vi "Test.vi"() -> ()   [LabVIEW 2020]
uses:
  Support/Controls/Cmd_Mouse Popup.ctl
  <vilib>/Utility/NIReport.llb/Report Type.ctl
  <vilib>/Utility/NIReport.llb/NI_report.lvclass
  <vilib>/Utility/NIReport.llb/Excel/NI_Excel.lvclass
  <vilib>/Utility/NIReport.llb/NI_ReportGenerationCore.lvlib
panel:
  in  "확인 버튼":bool
  in  "정지":bool
  in  "테이블 컨트롤":string[][](table)
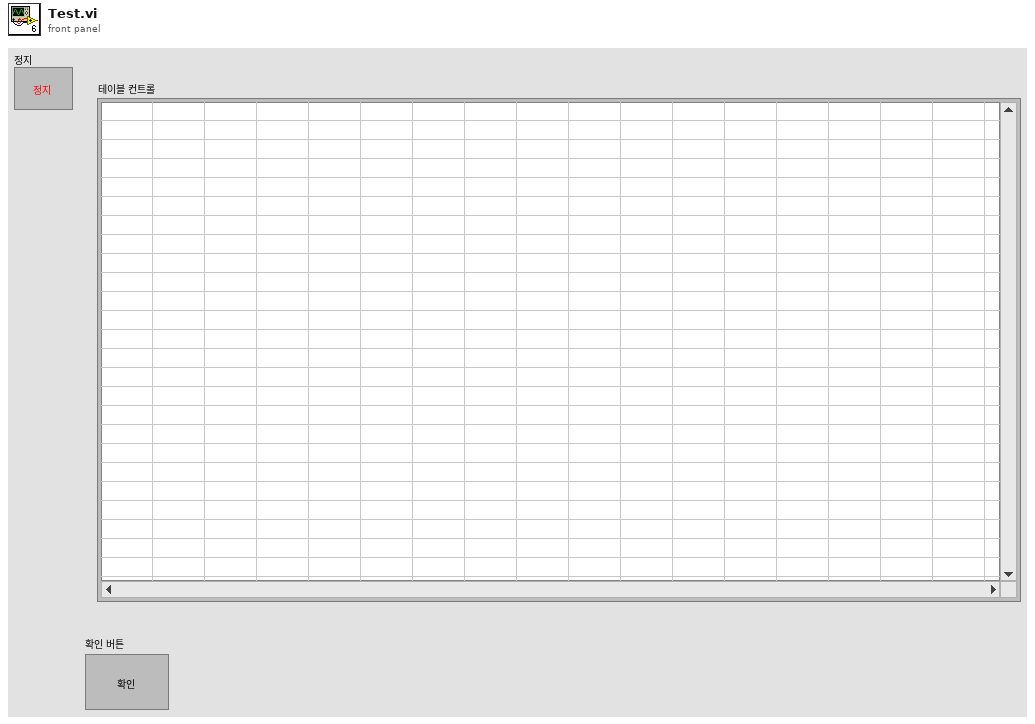
[diagram p1: front panel]
types:
  T1 = typedef "Cmd_Mouse Popup.ctl" = enum16{"활성화", "메뉴선택"}
  T2 = typedef "NI_ReportGenerationCore.lvlib/Report Type.ctl" = enum16{"HTML", "Word", "Excel"}
  T3 = enum16{"maximized", "minimized", "normal", "no change"}
  T4 = cluster{"Shift":bool, "Ctrl":bool, "Alt":bool, "Cmd":bool, "Opt":bool}
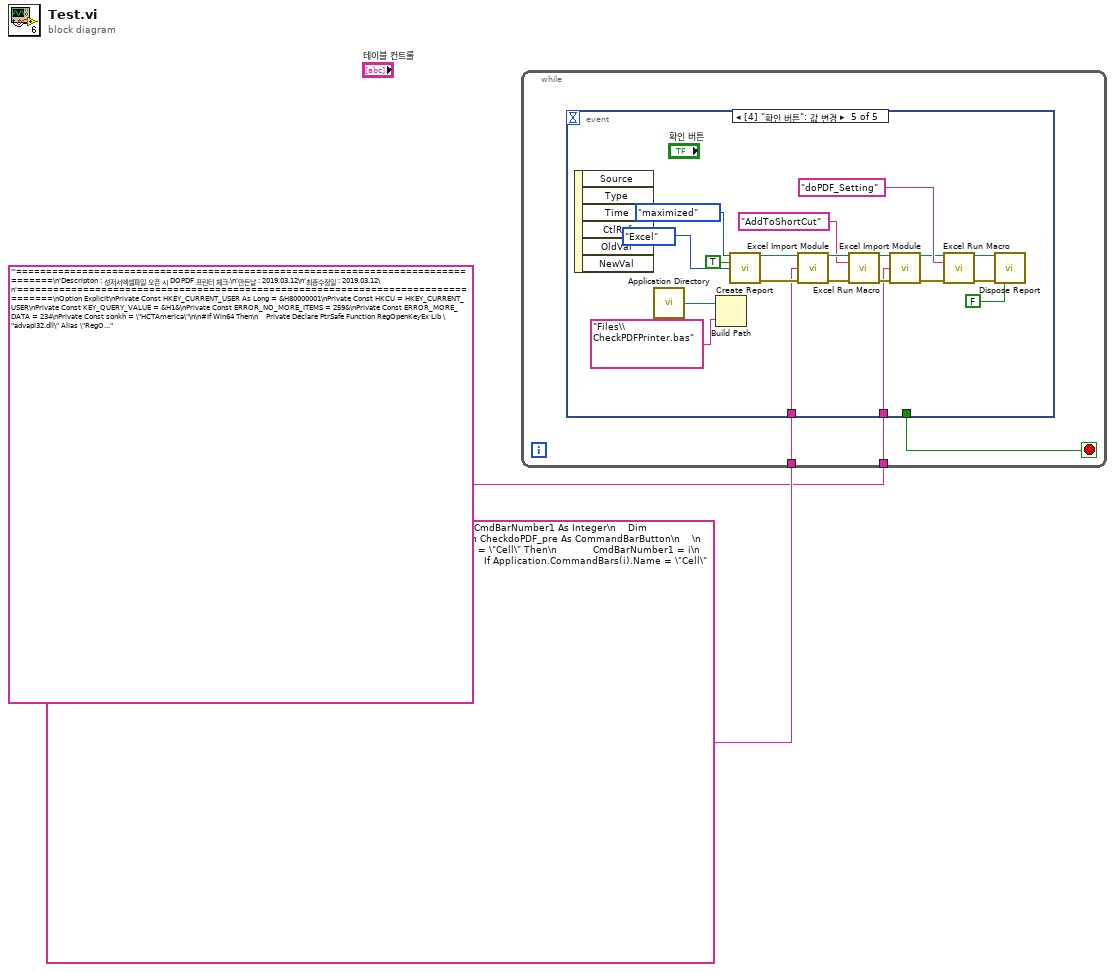
[diagram p0: block diagram]
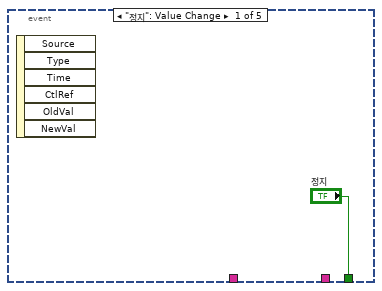
[diagram p2: hidden frame]
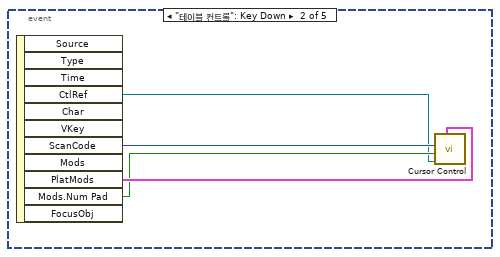
[diagram p3: hidden frame]
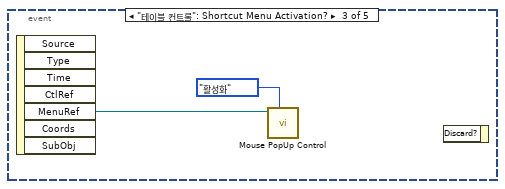
[diagram p4: hidden frame]
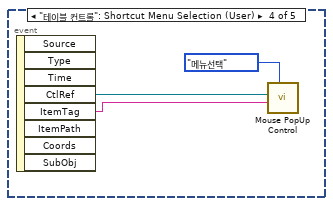
[diagram p5: hidden frame]
diagram:
  n1 = while {
    tunnel: "Sub AddToShortCut()\n\n    Dim i As Integer\n    Dim CmdBarNumber As Integer\n    Dim CmdBarNumber1 As Integer\n    Dim CmdBarNumber2 As Integer\n    Dim CheckdoPDF_preview As CommandBarButton\n    Dim CheckdoPDF_pre As CommandBarButton\n    \n    For i = 1 To Application.CommandBars.Count\n        If Application.CommandBars(i).Name = \"Cell\" Then\n            CmdBarNumber1 = i\n            Exit For\n        End If\n    Next\n\n    For i = 1 + i To Application.CommandBars.Count\n        If Application.CommandBars(i).Name = \"Cell\" Then\n            CmdBarNumber2 = i\n            Exit For\n        End If\n    Next\n\n    For i = 0 To 1\n\n        If i = 0 Then\n            CmdBarNumber = CmdBarNumber1\n        Else\n            CmdBarNumber = CmdBarNumber2\n        End If\n\n        With Application.CommandBars(CmdBarNumber)\n\n            .Reset\n            Set CheckdoPDF_preview = .Controls.Add(Type:=msoControlButton, Before:=8, Temporary:=True)\n            Set CheckdoPDF_pre = .Controls.Add(Type:=msoControlButton, Before:=9, Temporary:=True)\n            .Controls(10).BeginGroup = True\n\n        End With\n\n      \n        With CheckdoPDF_preview\n            .Caption = \"성적서출력확인(Preview)\"\n            .OnAction = \"xlPageBreakPreview_on\"\n            .FaceId = 487\n        End With\n        \n        With CheckdoPDF_pre\n            .Caption = \"성적서출력확인완료(업로드가능)\"\n            .OnAction = \"UpdatePreviewcheck\"\n            .FaceId = 487\n        End With\n        \n    Next\nEnd Sub\n" -> [w4]
    tunnel: "'==================================================================================\n'Descripton : 성저서엑셀파일 오픈 시 DOPDF 프린터 체크.\n'만든날 : 2019.03.12\n'최종수정일 : 2019.03.12\n'==================================================================================\nOption Explicit\nPrivate Const HKEY_CURRENT_USER As Long = &H80000001\nPrivate Const HKCU = HKEY_CURRENT_USER\nPrivate Const KEY_QUERY_VALUE = &H1&\nPrivate Const ERROR_NO_MORE_ITEMS = 259&\nPrivate Const ERROR_MORE_DATA = 234\nPrivate Const sonkh = \"HCTAmerica\"\n\n#If Win64 Then\n    Private Declare PtrSafe Function RegOpenKeyEx Lib \"advapi32.dll\" Alias \"RegOpenKeyExA\" ( _\n         ByVal hKey As LongPtr, _\n         ByVal lpSubKey As String, _\n         ByVal ulOptions As Long, _\n         ByVal samDesired As Long, _\n         phkResult As LongPtr) As Long\n  \n    Private Declare PtrSafe Function RegEnumValue Lib \"advapi32.dll\" Alias \"RegEnumValueA\" ( _\n          ByVal hKey As LongPtr, ByVal dwIndex As Long, ByVal lpValueName As String, _\n          lpcbValueName As Long, ByVal lpReserved As Long, lpType As Long, _\n          lpData As Byte, lpcbData As Long) As Long\n         \n    Private Declare PtrSafe Function RegCloseKey Lib \"advapi32.dll\" ( _\n         ByVal hKey As LongPtr) As Long\n     \n#Else\n    Private Declare Function RegOpenKeyEx Lib \"advapi32\" _\n        Alias \"RegOpenKeyExA\" ( _\n        ByVal hKey As Long, _\n        ByVal lpSubKey As String, _\n        ByVal ulOptions As Long, _\n        ByVal samDesired As Long, _\n        phkResult As Long) As Long\n    \n    Private Declare Function RegEnumValue Lib \"advapi32.dll\" _\n        Alias \"RegEnumValueA\" ( _\n        ByVal hKey As Long, _\n        ByVal dwIndex As Long, _\n        ByVal lpValueName As String, _\n        lpcbValueName As Long, _\n        ByVal lpReserved As Long, _\n        lpType As Long, _\n        lpData As Byte, _\n        lpcbData As Long) As Long\n    \n    Private Declare Function RegCloseKey Lib \"advapi32.dll\" ( _\n        ByVal hKey As Long) As Long\n    \n#End If\n    \nPrivate Function Crypt_EXcel(texti, salt) As String\n    Dim X1 As Long\n    Dim T, TT As Long\n    Dim G, sana As Long\n    Dim Crypted As String\n    \n  On Error Resume Next\n\n  For T = 1 To Len(salt)\n    sana = Asc(Mid(salt, T, 1))\n    X1 = X1 + sana\n  Next\n\n  X1 = Int((X1 * 0.1) / 6)\n  salt = X1\n  G = 0\n\n  For TT = 1 To Len(texti)\n    sana = Asc(Mid(texti, TT, 1))\n\n    G = G + 1\n\n    If G = 6 Then G = 0\n\n    X1 = 0\n\n    If G = 0 Then X1 = sana - (salt - 2)\n    If G = 1 Then X1 = sana + (salt - 5)\n    If G = 2 Then X1 = sana - (salt - 4)\n    If G = 3 Then X1 = sana + (salt - 2)\n    If G = 4 Then X1 = sana - (salt - 3)\n    If G = 5 Then X1 = sana + (salt - 5)\n\n    X1 = X1 + G\n\n    Crypted = Crypted & Chr(X1)\n\n  Next\n\n  Crypt_EXcel = Crypted\n\nEnd Function\nPrivate Function GetPrinterFullNames() As String()\nDim Printers() As String ' array of names to be returned\nDim PNdx As Long    ' index into Printers()\n'Dim hKey As Long    ' registry key handle\nDim Res As Long     ' result of API calls\nDim Ndx As Long     ' index for RegEnumValue\nDim ValueName As String ' name of each value in the printer key\nDim ValueNameLen As Long    ' length of ValueName\nDim DataType As Long        ' registry value data type\nDim ValueValue() As Byte    ' byte array of registry value value\nDim ValueValueS As String   ' ValueValue converted to String\nDim CommaPos As Long        ' position of comma character in ValueValue\nDim ColonPos As Long        ' position of colon character in ValueValue\nDim M As Long               ' string index\n\n#If Win64 Then\n    Dim L As LongPtr, hKey As LongPtr\n#Else\n    Dim L As Long, hKey As Long\n#End If\n\n' registry key in HCKU listing printers\nConst PRINTER_KEY = \"Software\\Microsoft\\Windows NT\\CurrentVersion\\Devices\"\n\nPNdx = 0\nNdx = 0\n' assume printer name is less than 256 characters\nValueName = String$(256, Chr(0))\nValueNameLen = 255\n' assume the port name is less than 1000 characters\nReDim ValueValue(0 To 999)\n' assume there are less than 1000 printers installed\nReDim Printers(1 To 1000)\n\n' open the key whose values enumerate installed printers\nRes = RegOpenKeyEx(HKCU, PRINTER_KEY, 0&, _\n    KEY_QUERY_VALUE, hKey)\n' start enumeration loop of printers\nRes = RegEnumValue(hKey, Ndx, ValueName, _\n    ValueNameLen, 0&, DataType, ValueValue(0), 1000)\n' loop until all values have been enumerated\nDo Until Res = ERROR_NO_MORE_ITEMS\n    M = InStr(1, ValueName, Chr(0))\n    If M > 1 Then\n        ' clean up the ValueName\n        ValueName = Left(ValueName, M - 1)\n    End If\n    ' find position of a comma and colon in the port name\n    CommaPos = InStr(1, ValueValue, \",\")\n    ColonPos = InStr(1, ValueValue, \":\")\n    ' ValueValue byte array to ValueValueS string\n    On Error Resume Next\n    ValueValueS = Mid(ValueValue, CommaPos + 1, ColonPos - CommaPos)\n    On Error GoTo 0\n    ' next slot in Printers\n    PNdx = PNdx + 1\n    Printers(PNdx) = ValueValueS & \"에 있는 \" & ValueName\n    ' reset some variables\n    ValueName = String(255, Chr(0))\n    ValueNameLen = 255\n    ReDim ValueValue(0 To 999)\n    ValueValueS = vbNullString\n    ' tell RegEnumValue to get the next registry value\n    Ndx = Ndx + 1\n    ' get the next printer\n    Res = RegEnumValue(hKey, Ndx, ValueName, ValueNameLen, _\n        0&, DataType, ValueValue(0), 1000)\n    ' test for error\n    If (Res <> 0) And (Res <> ERROR_MORE_DATA) Then\n        Exit Do\n    End If\nLoop\n' shrink Printers down to used size\nReDim Preserve Printers(1 To PNdx)\nRes = RegCloseKey(hKey)\n' Return the result array\nGetPrinterFullNames = Printers\nEnd Function\n\nSub doPDF_Setting()\n    Dim Printers() As String\n    Dim N As Long\n    Dim s As String\n    \n    On Error Resume Next\n    \n    Printers = GetPrinterFullNames()\n    For N = LBound(Printers) To UBound(Printers)\n        's = s & Printers(N) & vbNewLine\n    If InStr(1, Printers(N), \"doPDF\") > 1 Then '   If Trim(Mid(Printers(N), 11)) = \"doPDF 10\" Then\n            Application.ActivePrinter = Printers(N)\n            s = \"1\"\n        End If\n    Next N\n    If s <> \"1\" Then\n        If Mid(ActiveWorkbook.Name, 1, 4) <> \"C-20\" Then\n        Else\n            MsgBox \"doPDF가 없습니다. 확인 바랍니다.\" & vbCrLf & \"※성적서 업로드 전 미리보기확인 시 필요\" & vbCrLf & \"<게시판 참조-교정사업부-CAMAS에러및개선>\", vbOKOnly, \"HCT_Calibratoin_QA\"\n\n        End If\n    End If\n    \nEnd Sub\n\nFunction doPDF_Setting_recheck() As Boolean\n    Dim Printers() As String\n    Dim N As Long\n    Dim s As String\n    \n    On Error Resume Next\n    \n    Printers = GetPrinterFullNames()\n    For N = LBound(Printers) To UBound(Printers)\n        's = s & Printers(N) & vbNewLine\n        If InStr(1, Printers(N), \"doPDF\") > 1 Then '        If Trim(Mid(Printers(N), 11)) = \"doPDF 10\" Then\n            Application.ActivePrinter = Printers(N)\n            s = \"1\"\n        End If\n    Next N\n    If s <> \"1\" Then\n        If Mid(ActiveWorkbook.Name, 1, 4) <> \"C-20\" Then\n        Else\n            MsgBox \"재확인!doPDF가 없습니다. 확인 바랍니다.\" & vbCrLf & \"※성적서 업로드 전 미리보기확인 시 필요\" & vbCrLf & \"<게시판 참조-교정사업부-CAMAS에러및개선>\", vbOKOnly, \"HCT_Calibratoin_QA\"\n            doPDF_Setting_recheck = False\n            Exit Function\n        End If\n    End If\n    doPDF_Setting_recheck = True\nEnd Function\n\n\nSub xlPageBreakPreview_on()\n    Dim page2_01 As Integer\n    Dim first_page As Integer\n    Dim I_Cnt As Integer\n    \n    Dim sheets_PrintQuality1 As Integer\n    Dim sheets_PrintQuality2 As Integer\n    \n    If Mid(ActiveWorkbook.Name, 1, 4) <> \"C-20\" Then\n        Exit Sub\n    End If\n    \n    If doPDF_Setting_recheck = False Then\n        MsgBox \"doPDF 설치바랍니다.\" & vbCrLf & \"※미설치 시 진행 안됨\" & vbCrLf & \"<게시판 참조-교정사업부-CAMAS에러및개선>\", vbOKOnly, \"HCT_Calibratoin_QA\"\n        \n        Exit Sub\n    End If\n    first_page = 0\n    page2_01 = 0\n    \n    '기존처리와 동일하게하기위해서 처리\n    sheets_PrintQuality1 = Application.Worksheets(\"교정결과\").PageSetup.PrintQuality(1)\n    sheets_PrintQuality2 = Application.Worksheets(\"교정결과\").PageSetup.PrintQuality(2)\n    Application.Worksheets(\"교정결과\").PageSetup.HeaderMargin = 0 ' 페이지설정-여백-머릿글\n    Application.Worksheets(\"교정결과\").PageSetup.FooterMargin = 0  ' 페이지설정-여백-바닥글\n    Application.Worksheets(\"교정결과\").PageSetup.CenterHorizontally = True\n     \n     '=====================\n    If sheets_PrintQuality1 < sheets_PrintQuality2 Then\n        sheets_PrintQuality1 = sheets_PrintQuality2\n    End If\n    \n    If sheets_PrintQuality1 <> 300 And sheets_PrintQuality1 <> 600 And sheets_PrintQuality1 <> 1200 Then\n        sheets_PrintQuality1 = 600\n    End If\n    '=====================\n    \n    \n    \n    For I_Cnt% = 1 To Application.Sheets.Count\n        If Application.Sheets(I_Cnt%).Name = \"교정결과2\" Then\n            page2_01 = page2_01 + 1\n            Application.Sheets(I_Cnt%).DisplayAutomaticPageBreaks = True\n            Application.Sheets(I_Cnt%).PageSetup.PrintQuality = sheets_PrintQuality1\n            ActiveWindow.View = xlPageBreakPreview\n        End If\n        If Application.Sheets(I_Cnt%).Name = \"부록\" Then\n            page2_01 = page2_01 + 2\n            Application.Sheets(I_Cnt%).DisplayAutomaticPageBreaks = True\n            Application.Sheets(I_Cnt%).PageSetup.PrintQuality = sheets_PrintQuality1\n            ActiveWindow.View = xlPageBreakPreview\n        End If\n        If Application.Sheets(I_Cnt%).Name = \"판정결과\" Then\n            page2_01 = page2_01 + 4\n            Application.Sheets(I_Cnt%).DisplayAutomaticPageBreaks = True\n            Application.Sheets(I_Cnt%).PageSetup.PrintQuality = sheets_PrintQuality1\n            ActiveWindow.View = xlPageBreakPreview\n        End If\n        If Application.Sheets(I_Cnt%).Name = \"부록2\" Then\n            page2_01 = page2_01 + 8\n            Application.Sheets(I_Cnt%).DisplayAutomaticPageBreaks = True\n            Application.Sheets(I_Cnt%).PageSetup.PrintQuality = sheets_PrintQuality1\n            ActiveWindow.View = xlPageBreakPreview\n        End If\n        If Application.Sheets(I_Cnt%).Name = \"교정결과\" Then\n            Application.Sheets(I_Cnt%).DisplayAutomaticPageBreaks = True\n            Application.Sheets(I_Cnt%).PageSetup.PrintQuality = sheets_PrintQuality1\n            ActiveWindow.View = xlPageBreakPreview\n        End If\n        If Application.Sheets(I_Cnt%).Name = \"한글성적서\" Then\n            first_page = 100\n            Application.Sheets(I_Cnt%).DisplayAutomaticPageBreaks = True\n            Application.Sheets(I_Cnt%).PageSetup.PrintQuality = sheets_PrintQuality1\n            ActiveWindow.View = xlPageBreakPreview\n        End If\n        \n    Next\n    \n    Select Case page2_01 + first_page\n        Case 0\n            Application.Worksheets(Array(\"교정결과\")).Select\n        Case 1\n            Application.Worksheets(Array(\"교정결과\", \"교정결과2\")).Select\n        Case 2\n            Application.Worksheets(Array(\"교정결과\", \"부록\")).Select\n        Case 3\n            Application.Worksheets(Array(\"교정결과\", \"교정결과2\", \"부록\")).Select\n        Case 4\n            Application.Worksheets(Array(\"교정결과\", \"판정결과\")).Select\n        Case 5\n            Application.Worksheets(Array(\"교정결과\", \"교정결과2\", \"판정결과\")).Select\n        Case 6\n            Application.Worksheets(Array(\"교정결과\", \"부록\", \"판정결과\")).Select\n        Case 7\n            Application.Worksheets(Array(\"교정결과\", \"교정결과2\", \"부록\", \"판정결과\")).Select\n                                \n        Case 8\n            Application.Worksheets(Array(\"교정결과\", \"부록2\")).Select\n        Case 9\n            Application.Worksheets(Array(\"교정결과\", \"교정결과2\", \"부록2\")).Select\n        Case 10\n            Application.Worksheets(Array(\"교정결과\", \"부록\", \"부록2\")).Select\n        Case 11\n            Application.Worksheets(Array(\"교정결과\", \"교정결과2\", \"부록\", \"부록2\")).Select\n        Case 12\n            Application.Worksheets(Array(\"교정결과\", \"부록2\", \"판정결과\")).Select\n        Case 13\n            Application.Worksheets(Array(\"교정결과\", \"교정결과2\", \"부록2\", \"판정결과\")).Select\n        Case 14\n            Application.Worksheets(Array(\"교정결과\", \"부록\", \"부록2\", \"판정결과\")).PrintOut\n        Case 15\n            Application.Worksheets(Array(\"교정결과\", \"교정결과2\", \"부록\", \"부록2\", \"판정결과\")).Select\n                    \n                    \n        Case 100\n            Application.Worksheets(Array(\"한글성적서\", \"교정결과\")).Select\n        Case 101\n            Application.Worksheets(Array(\"한글성적서\", \"교정결과\", \"교정결과2\")).Select\n        Case 102\n            Application.Worksheets(Array(\"한글성적서\", \"교정결과\", \"부록\")).Select\n        Case 103\n            Application.Worksheets(Array(\"한글성적서\", \"교정결과\", \"교정결과2\", \"부록\")).Select\n        Case 104\n            Application.Worksheets(Array(\"한글성적서\", \"교정결과\", \"판정결과\")).Select\n        Case 105\n            Application.Worksheets(Array(\"한글성적서\", \"교정결과\", \"교정결과2\", \"판정결과\")).Select\n        Case 106\n            Application.Worksheets(Array(\"한글성적서\", \"교정결과\", \"부록\", \"판정결과\")).Select\n        Case 107\n            Application.Worksheets(Array(\"한글성적서\", \"교정결과\", \"교정결과2\", \"부록\", \"판정결과\")).Select\n                                \n        Case 108\n            Application.Worksheets(Array(\"한글성적서\", \"교정결과\", \"부록2\")).Select\n        Case 109\n            Application.Worksheets(Array(\"한글성적서\", \"교정결과\", \"교정결과2\", \"부록2\")).Select\n        Case 110\n            Application.Worksheets(Array(\"한글성적서\", \"교정결과\", \"부록\", \"부록2\")).Select\n        Case 111\n            Application.Worksheets(Array(\"한글성적서\", \"교정결과\", \"교정결과2\", \"부록\", \"부록2\")).Select\n        Case 112\n            Application.Worksheets(Array(\"한글성적서\", \"교정결과\", \"부록2\", \"판정결과\")).Select\n        Case 113\n            Application.Worksheets(Array(\"한글성적서\", \"교정결과\", \"교정결과2\", \"부록2\", \"판정결과\")).Select\n        Case 114\n            Application.Worksheets(Array(\"한글성적서\", \"교정결과\", \"부록\", \"부록2\", \"판정결과\")).PrintOut\n        Case 115\n            Application.Worksheets(Array(\"한글성적서\", \"교정결과\", \"교정결과2\", \"부록\", \"부록2\", \"판정결과\")).Select\n            \n            \n    End Select\n    \n    ActiveWindow.SelectedSheets.PrintPreview\n    Application.Sheets(\"교정결과\").Select\n\nEnd Sub\nSub UpdatePreviewcheck()\n\n    Dim s As Worksheet\n        \n    If Mid(ActiveWorkbook.Name, 1, 4) <> \"C-20\" Then\n        Exit Sub\n    End If\n    \n    If doPDF_Setting_recheck = False Then\n        MsgBox \"doPDF 설치바랍니다.\" & vbCrLf & \"※미설치 시 진행 안됨\", vbOKOnly, \"HCT_Calibratoin_QA\"\n        \n        Exit Sub\n    End If\n    \n    For Each s In Worksheets\n        s.DisplayAutomaticPageBreaks = True\n        If s.Name = \"기본정보\" Then\n            s.Activate\n            s.Cells(49, 1).Value = Crypt_EXcel(s.Cells(3, 8).Value, sonkh) '20190313 정현진CJ MCT 협의완료\n            \n        End If\n    Next\n\nEnd Sub\n" -> [w3]
    stop <- w5 stop-if-true
    n2 = event shown="[4] \"확인 버튼\": 값 변경" {
      selector: _ -> [_ _ _ _ _]
      dyn-events: _ -> [_ _ _ _ _]
      timeout: _ -> [_ _ _ _ _]
      tunnel: ["정지" _ _ _ _] -> w5
      tunnel: w4 -> [_ _ _ _ w22]
      tunnel: w3 -> [_ _ _ _ w17]
      event "정지": Value Change {
        n3 = event-data() -> ()  [unwired: 1 in, 6 out]
      }
      event "테이블 컨트롤": Key Down {
        n4 = event-data() -> ("CtlRef"=w7:refnum<vi>, "ScanCode"=w9:i16, "PlatMods"=w10:T4, "Mods.Num Pad"=w8:bool)  [unwired: 1 in, 7 out]
        n5 = call "Cursor Control.vi"("플랫폼 조합키"=w10, "참조"=w7, "Num Pad"=w8, "ScanCode"=w9) -> ()  [unwired: 6 in, 2 out]
      }
      event "테이블 컨트롤": Shortcut Menu Activation? {
        n6 = event-data() -> ("MenuRef"=w11:refnum<k9>)  [unwired: 1 in, 6 out]
        n7 = call "Mouse PopUp Control.vi"("type"=Cmd_Mouse_Popup."활성화", "메뉴 참조"=w11) -> ()  [unwired: 9 in, 1 out]
        n8 = event-data() -> ()  [unwired: 2 in, 1 out]
      }
      event "테이블 컨트롤": Shortcut Menu Selection (User) {
        n9 = event-data() -> ("CtlRef"=w14:refnum<vi>, "ItemTag"=w13:string)  [unwired: 1 in, 6 out]
        n10 = call "Mouse PopUp Control.vi"("type"=Cmd_Mouse_Popup."메뉴선택", "아이템 태그"=w13, "Tbl 참조 번호"=w14) -> ()  [unwired: 8 in, 1 out]
      }
      event "확인 버튼": Value Change {
        n11 = event-data() -> ()  [unwired: 1 in, 6 out]
        n12 = call <vilib>:"Application Directory.vi"() -> ("Application Directory"=w32:path)
        n13 = Build Path(base path=w32, name or relative path="Files\\CheckPDFPrinter.bas" ("이름 또는 상대 경로")) -> ()  [unwired: 1 out]
        n14 = call <vilib>:"Create Report.vi"("window state (normal)"=T3."maximized", "display alerts? (F)"=TRUE, "report type"=Report_Type."Excel") -> ("report out"=w35:refnum<class "NI_report.lvclass">, "error out"=w34:errorcluster)  [unwired: 11 in]
        n15 = call <vilib>:"Excel Import Module.vi"("report in"=w35, "module code (\"\")"=w22, "error in (no error)"=w34) -> ("report out"=w25:refnum<class "NI_report.lvclass">, "error out"=w26:errorcluster)  [unwired: 10 in, 1 out]
        n16 = call <vilib>:"Excel Run Macro.vi"("report in"=w25, "macro name"="AddToShortCut", "error in (no error)"=w26) -> ("report out"=w21:refnum<class "NI_report.lvclass">, "error out"=w20:errorcluster)  [unwired: 10 in, 1 out]
        n17 = call <vilib>:"Excel Import Module.vi"("report in"=w21, "module code (\"\")"=w17, "error in (no error)"=w20) -> ("report out"=w19:refnum<class "NI_report.lvclass">, "error out"=w18:errorcluster)  [unwired: 10 in, 1 out]
        n18 = call <vilib>:"Excel Run Macro.vi"("report in"=w19, "macro name"="doPDF_Setting", "error in (no error)"=w18) -> ("report out"=w24:refnum<class "NI_report.lvclass">, "error out"=w28:errorcluster)  [unwired: 10 in, 1 out]
        n19 = call-dynamic "Dispose Report.vi"("report in"=w24, "error in (no error)"=w28, "close report? (T)"=FALSE) -> ()  [unwired: 12 in, 1 out]
      }
    }
  }
